vi "Module ID.vi"(11 "System Status Module in":refnum<class "System Status Module.lvclass">) -> (2 "Module ID":string)   [LabVIEW 2020, in "VolatusGUI.lvlib" / "System Status Module.lvclass"]
uses:
  System Status Module.lvclass
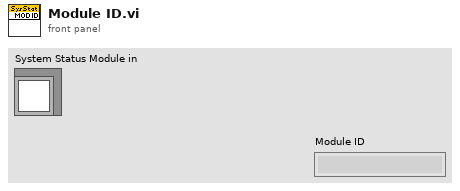
[diagram p1: front panel]
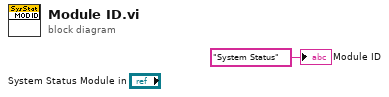
[diagram p0: block diagram]
diagram:
  "Module ID" <- "System Status" ("Module ID")
